vi "emitters to PDWs.vi"(0 "emmiter":T3[](array[typedef]) {"t end" format="%#_3p"; "t start" format="%#_3p"; "DOA" format="%#_3p"}, 9 "center frequency (Hz)":dbl=1.0 format="%.2f", 11 "erorr in":errorcluster) -> (4 "sorted array":T1[](array[typedef]), 10 "may saturate":bool, 15 "erorr out":errorcluster)   [LabVIEW 2021]
uses:
  02974b87-4f9c-4a39-b6ec-6068b831107f.vi
  mode_type.ctl
  PDW_lv2.ctl
  emitter params.ctl
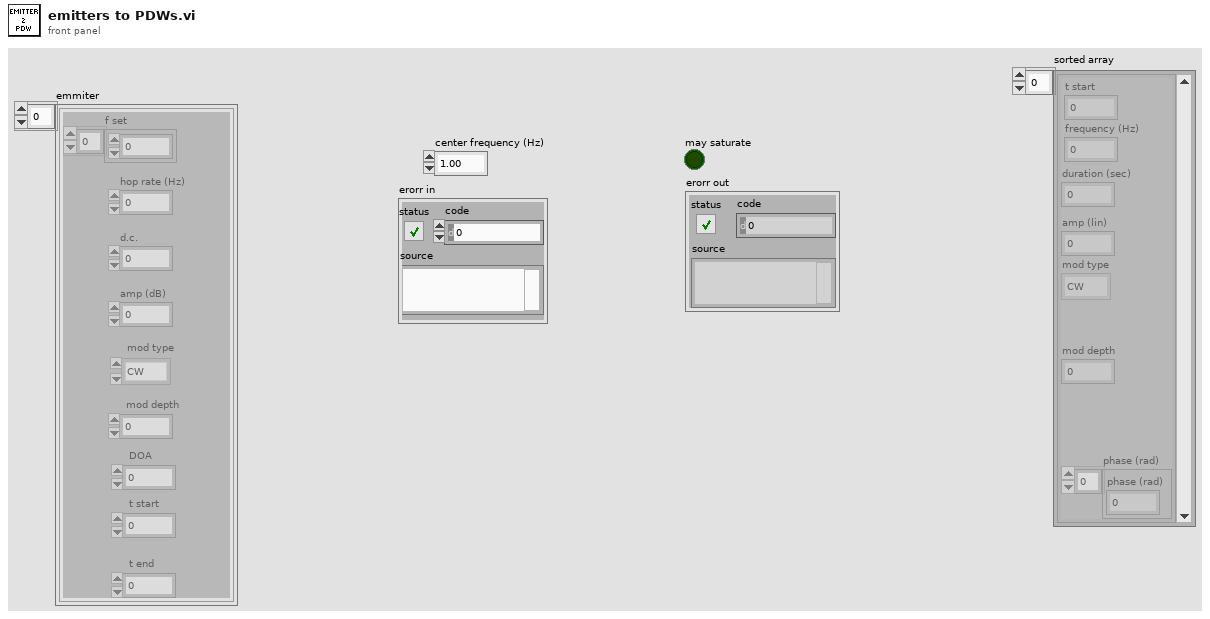
[diagram p1: front panel]
types:
  T1 = typedef "PDW_lv2.ctl" = cluster{"t start":dbl, "frequency (Hz)":dbl, "duration (sec)":dbl, "amp (lin)":dbl, "mod type":T2, "mod depth":dbl, "phase (rad)":dbl[]}
  T2 = typedef "mode_type.ctl" = enum8{"CW", "NC - CW", "NC - cw", "LFM", "BPSK", "QPSK"}
  T3 = typedef "emitter params.ctl" = cluster{"f set":dbl[], "hop rate (Hz)":dbl, "d.c.":dbl, "amp (dB)":dbl, "mod type":T2, "mod depth":dbl, "DOA":dbl, "t start":dbl, "t end":dbl}
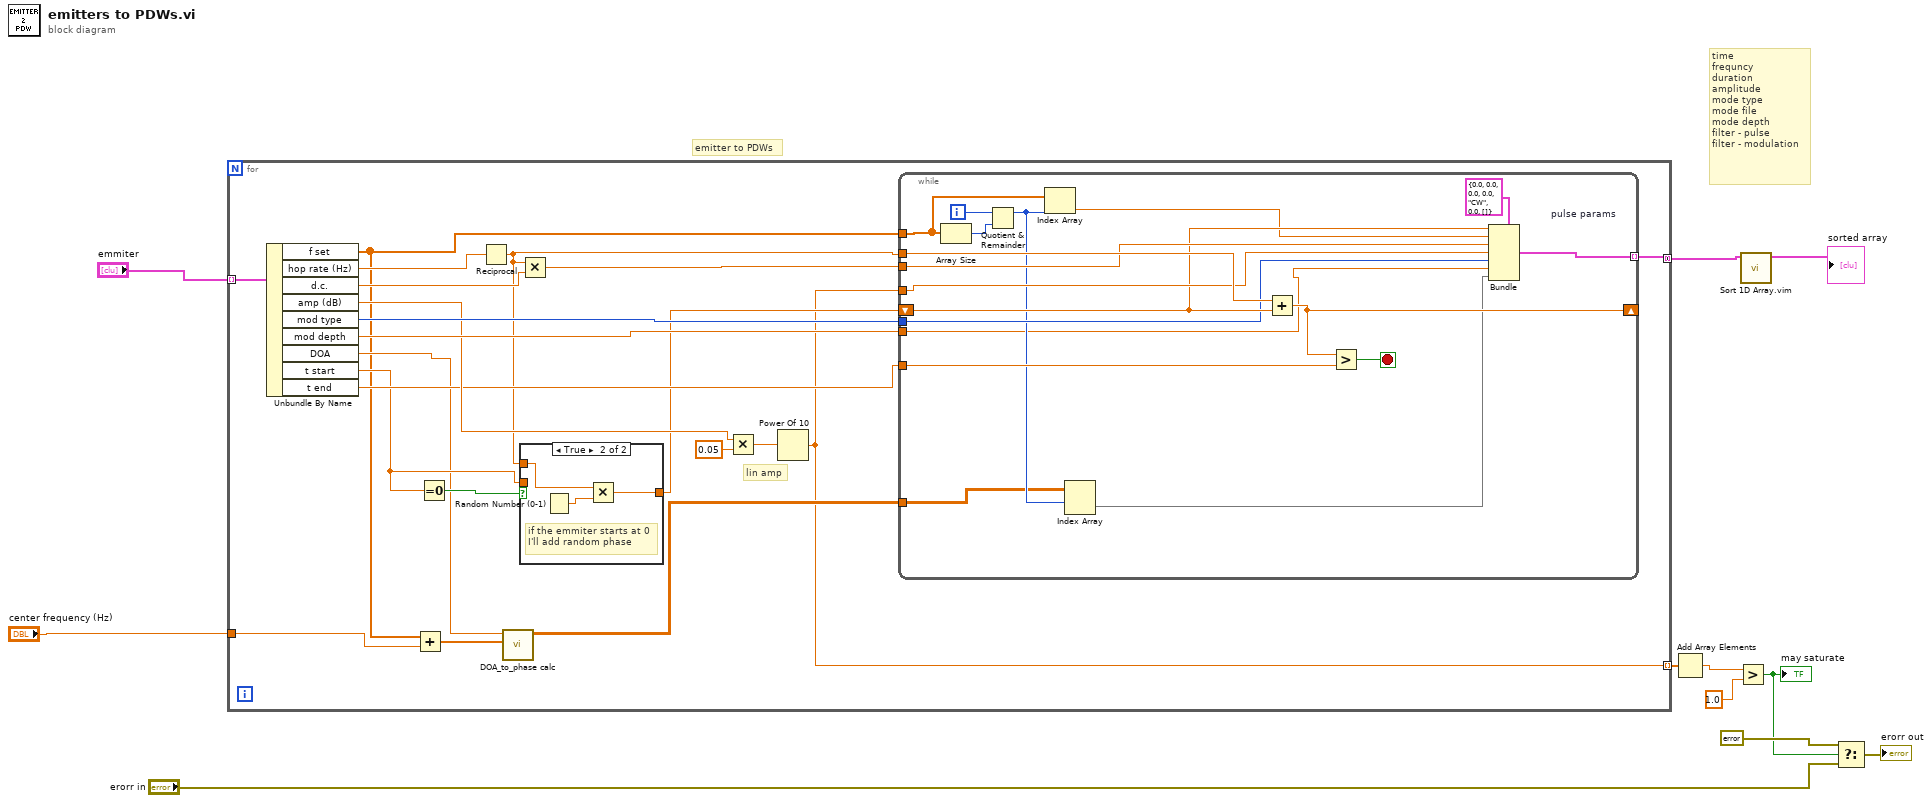
[diagram p0: block diagram]
diagram:
  # "time\nfrequncy\nduration\namplitude\nmode type\nmode file\nmode depth\nfilter - pulse\nfilter - modulation"
  # "emitter to PDWs"
  n1 = for {
    tunnel: "emmiter" -> [w32] mode=indexing
    tunnel: [w29] -> w11 mode=concatenating
    tunnel: "center frequency (Hz)" -> [w15]
    tunnel: [w12] -> w8 mode=indexing
    # "lin amp"
    n2 = Unbundle By Name(w32) -> ("f set"=w16:dbl[], "hop rate (Hz)"=w26:dbl, "d.c."=w31:dbl, "amp (dB)"=w23:dbl, "mod type"=w28:T2, "mod depth"=w27:dbl, "DOA"=w17:dbl, "t start"=w18:dbl, "t end"=w22:dbl)
    n3 = Add(x=w16, y=w15) -> (x+y=w14:dbl[])
    n4 = Equal To 0?(x=w18) -> (x = 0?=w20:bool)
    n5 = Reciprocal(x=w26) -> (1/x=w21:dbl)
    n6 = call "DOA_to_phase calc.vi"("f set (Hz)"=w14, "DOA (deg)"=w17) -> ("phase (rad)"=w13:dbl[][])  [unwired: 9 in]
    n7 = Multiply(x=w21, y=w31) -> (x*y=w30:dbl)
    n8 = case shown="True" w20 {
      tunnel: w21 -> [_ w35]
      tunnel: [w33 w34] -> w19
      tunnel: w18 -> [w33 _]
      frame False {
      }
      frame True {
        # "if the emmiter starts at 0\nI'll add random phase"
        n9 = Random Number (0-1)() -> (number: 0 to 1=w36:dbl)
        n10 = Multiply(x=w35, y=w36) -> (x*y=w34:dbl)
      }
    }
    n11 = Multiply(x=w23, y=0.05) -> (x*y=w24:dbl)
    n12 = Power Of 10(x=w24) -> (10^x=w12:dbl)
    n13 = while {
      tunnel: w16 -> [w52]
      shift-right: [w49] -> _
      shift-left: w19 -> [w44]
      tunnel: w21 -> [w51]
      tunnel: w22 -> [w50]
      tunnel: w30 -> [w47]
      tunnel: w12 -> [w46]
      tunnel: [w45] -> w29 mode=indexing
      tunnel: w28 -> [w42]
      tunnel: w27 -> [w37]
      tunnel: w13 -> [w40]
      i -> [w54]
      stop <- w48 stop-if-true
      n14 = Array Size(array=w52) -> (size(s)=w53:i32)
      n15 = Quotient & Remainder(x=w54, y=w53) -> (x-y*floor(x/y)=w41:i32)  [unwired: 1 out]
      n16 = Index Array(array=w52, index=w41) -> (element=w43:dbl)
      n17 = Index Array(array=w40, index (row)=w41) -> (element=w38:dbl[])  [unwired: 1 in]
      n18 = Add(x=w51, y=w44) -> (x+y=w49:dbl)
      n19 = Greater?(x=w49, y=w50) -> (0:w48:bool)
      n20 = Bundle "pulse params"(cluster=T1 {"t start"=0.0, "frequency (Hz)"=0.0, "duration (sec)"=0.0, "amp (lin)"=0.0, "mod type"=enum."CW", "mod depth"=0.0, "phase (rad)"=[]} ("Cluster"), "t start"=w44, "frequency (Hz)"=w43, "duration (sec)"=w47, "amp (lin)"=w46, "mod type"=w42, "mod depth"=w37, "phase (rad)"=w38) -> (w45:T1)
    }
  }
  n21 = Add Array Elements(numeric array=w8) -> (sum=w7:dbl)
  n22 = Greater?(x=w7, y=1.0) -> (0:w3:bool)
  "may saturate" <- w3
  n23 = call "Sort 1D Array.vim"("unsorted array"=w11) -> ("sorted array"=→"sorted array":T1[])  [unwired: 10 in]
  n24 = Select(t=errorcluster {"status"=FALSE, "code"=5432, "source"="the total amp of all the emmiters are higher then 1, if thay transmit togeder the output will saturate"} ("error out"), s=w3, f="erorr in") -> (s? t:f=→"erorr out":errorcluster)
